vi "reprGraphical.vi"(8 "error in (no error)":errorcluster, 9 "Image Descriptor":T1={"Upper-Left Corner Coordinates"={"UTM Zone"=0.0, "Hemisphere"=enum."North", "East"=0.0, "North"=0.0}, "Meters/Pixel"=42.294203} {"Upper-Left Corner Coordinates"."North" format="%#_10f"; "Upper-Left Corner Coordinates"."East" format="%#_8f"}, 10 "Image In":T3, 11 "Drive in":refnum<class "DriveTo.lvclass">) -> (0 "error out":errorcluster, 2 "Image Out":T3, 3 "Drive out":refnum<class "DriveTo.lvclass">)   [LabVIEW 2011, in "DriveTo.lvclass"]
uses:
  DriveTo.lvclass
  <vilib>/vision/Image Controls.llb/IMAQ Image.ctl
  0-OCU/0 Code/mission input/0-Image Descriptor.ctl
  2 Typedefs/UTM Location.ctl
  0x2-OCU-Think Comm/0x2 Typedefs/waypointTypes.ctl
  DriveTo.lvclass/DriveTo.ctl
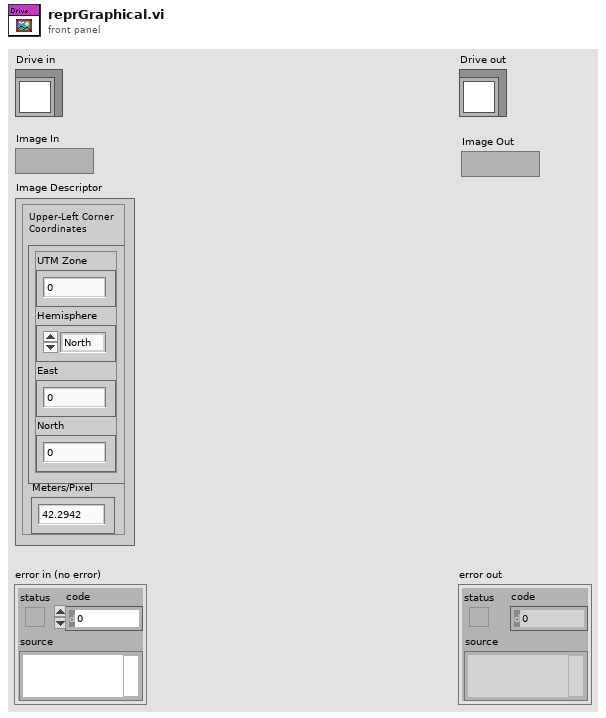
[diagram p1: front panel]
types:
  T1 = typedef "0-Image Descriptor.ctl" = cluster{"Upper-Left Corner Coordinates":T2, "Meters/Pixel":dbl}
  T2 = typedef "UTM Location.ctl" = cluster{"UTM Zone":dbl, "Hemisphere":enum16{"North", "South"}, "East":dbl, "North":dbl}
  T3 = typedef "IMAQ Image.ctl" = refnum<image>
  T4 = typedef "waypointTypes.ctl" = enum16{"Drive", "Round Port", "Round Starboard", "Stay"}
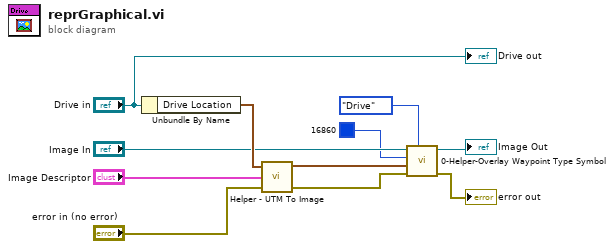
[diagram p0: block diagram]
diagram:
  n1 = Unbundle By Name("Drive in") -> ("Drive Location"=w11:T2)
  n2 = call "Helper - UTM To Image.vi"("error in"="error in (no error)", "Image Descriptor"="Image Descriptor", "UTM Location"=w11) -> ("error out"=w5:errorcluster, "Pixel Coordinates"=w4:cluster{"X":i32, "Y":i32})  [unwired: 1 out]
  n3 = call "0-Helper-Overlay Waypoint Type Symbol.vi"("Icon Type"=waypointTypes."Drive", "error in"=w5, "Overlay Location"=w4, "Icon Color"=u32 16860, "Image in"="Image In") -> ("error out"=→"error out":errorcluster, "Image out"=→"Image Out":T3)  [unwired: 5 in]
  "Drive out" <- "Drive in"
